vi "test_Retrieve Data From FPGA.vi"(8 "error in (no error)":errorcluster, 11 "Data from FIFO":u64[](array[numeric])=[5631702913073631, 5629503829180420, 5629508124147720, 5629503829180426, 5629508124147722, 5629503829180426, 5629508124147722, 5629503829180426, 5629508124147722, 5631707147403291]) -> (0 "error out":errorcluster, 3 "Queue Elements":T1[](array[typedef]))   [LabVIEW 2016]
uses:
  Host/Typedefs/Monitor Data Element.ctl
  Host/Typedefs/LV2G Operation.ctl
  Host/Typedefs/IO Buffer Operation.ctl
  Host/Typedefs/Monitor Data Operation.ctl
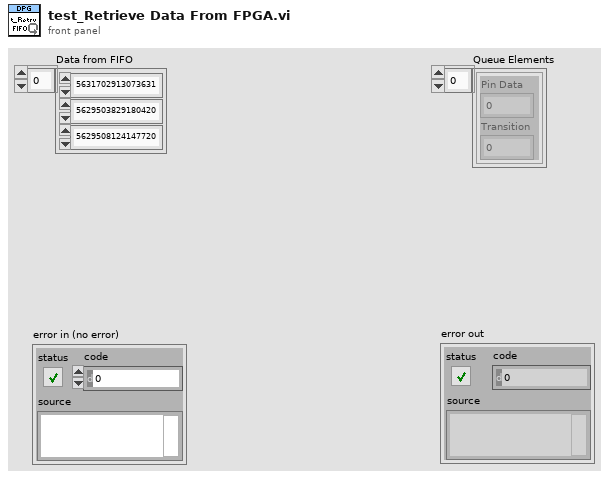
[diagram p1: front panel]
types:
  T1 = typedef "Monitor Data Element.ctl" = cluster{"Pin Data":u32, "Transition ":u32}
  T2 = typedef "IO Buffer Operation.ctl" = enum16{"Initialize", "Write IO Data_Rd", "Read IO Data_Rd", "Write IO Data_Wr", "Read IO Data_Wr", "Write  IO Data_Dir", "Read  IO Data_Dir", "Write Host to Target FIFO", "Read Host to Target FIFO", "Write Target to Host FIFO", "Read Target to Host FIFO", "Write Monitor Enable?", "Read Monitor Enable?", "Close"}
  T3 = typedef "LV2G Operation.ctl" = enum16{"Initialize", "Set", "Get", "Close"}
  T4 = typedef "Monitor Data Operation.ctl" = enum16{"Obtain", "Enqueue", "Read Elements", "Flush", "Release", "Read Last Element"}
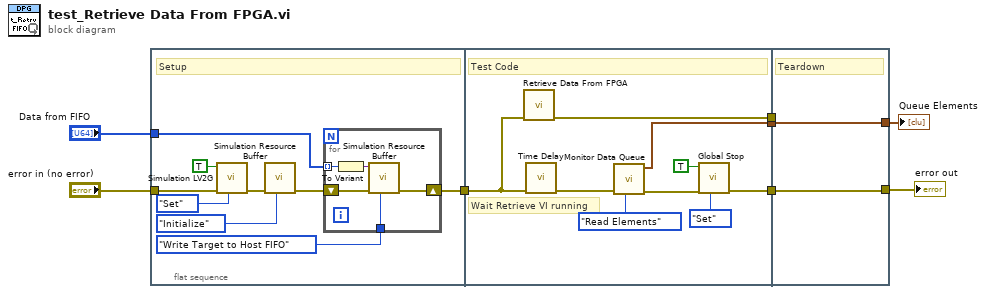
[diagram p0: block diagram]
diagram:
  n1 = flat-sequence {
    tunnel: "error in (no error)" -> [w17]
    tunnel: [w10] -> w8
    tunnel: "Data from FIFO" -> [w9]
    tunnel: w8 -> [w28]
    tunnel: [w31] -> w7
    tunnel: [w24] -> w4
    tunnel: [w23] -> w1
    tunnel: [w33] -> w5
    tunnel: w7 -> [w33]
    tunnel: w4 -> [w32]
    tunnel: [w32] -> w3
    tunnel: w1 -> [_]
    frame #0 {
      # "Setup"
      n2 = call "Simulation LV2G.vi"("Operation (Get)"=LV2G_Operation."Set", "error in (no error)"=w17, "Simulation?"=TRUE) -> ("error out"=w13:errorcluster)  [unwired: 7 in, 1 out]
      n3 = call "Simulation Resource Buffer.vi"("IO Buffer Operation"=IO_Buffer_Operation."Initialize", "error in (no error)"=w13) -> ("error out"=w12:errorcluster)  [unwired: 7 in, 2 out]
      n4 = for {
        tunnel: IO_Buffer_Operation."Write Target to Host FIFO" ("IO Buffer Operation") -> [w22]
        shift-right: [w19] -> w10
        shift-left: w12 -> [w20]
        tunnel: w9 -> [w18] mode=indexing
        n5 = To Variant(anything=w18) -> (Variant=w21:variant)
        n6 = call "Simulation Resource Buffer.vi"("IO Buffer Operation"=w22, "error in (no error)"=w20, "Data in"=w21) -> ("error out"=w19:errorcluster)  [unwired: 6 in, 2 out]
      }
    }
    frame #1 {
      # "Wait Retrieve VI running"
      # "Test Code"
      n7 = call "Retrieve Data From FPGA.vi"("error in (no error)"=w28) -> ("error out"=w23:errorcluster)  [unwired: 10 in]
      n8 = call "Time Delay"("error in (no error)"=w28) -> ("error out"=w26:errorcluster)  [unwired: 10 in]
      n9 = call "Monitor Data Queue.vi"("Queue Function"=Monitor_Data_Operation."Read Elements", "error in (no error)"=w26) -> ("error out"=w25:errorcluster, "Queue Elements"=w24:T1[])  [unwired: 6 in, 2 out]
      n10 = call "Global Stop.vi"("Stop Operation (Get)"=LV2G_Operation."Set", "error in (no error)"=w25, "Stop?"=TRUE) -> ("error out"=w31:errorcluster)  [unwired: 7 in, 1 out]
    }
    frame #2 {
      # "Teardown"
    }
  }
  "error out" <- w5
  "Queue Elements" <- w3
